vi "StreamCluster.vi"() -> ()   [LabVIEW 2024]
uses:
  Control/streamIO_states.ctl
  Control/StreamCluster_TypeDef.ctl
panel:
  in  "StreamCluster":T1
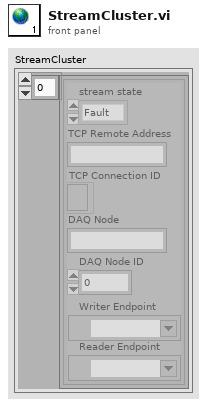
[diagram p1: front panel]
types:
  T1 = typedef "StreamCluster_TypeDef.ctl" = cluster{cluster{"stream state":T2, "TCP Remote Address":string, "TCP Connection ID":refnum<k5>, "DAQ Node":string, "DAQ Node ID":i32, "Writer Endpoint":refnum<k21>, "Reader Endpoint":refnum<k21>}[]}
  T2 = typedef "streamIO_states.ctl" = enum16{"Fault", "Initilize", "Stream", "Close"}
diagram:
